vi "hash action stack -- test.vi"() -> ()   [LabVIEW 2012]
uses:
  hash action control.ctl
  stack action -- control.ctl
panel:
  in  "hash action list":T1[](array[typedef])
  out "cursor window action out":T1
  out "stack is empty ?":bool
  in  "hash action":T1
  in  "stack action":T2
  in  "command stack":T1[](array[typedef])
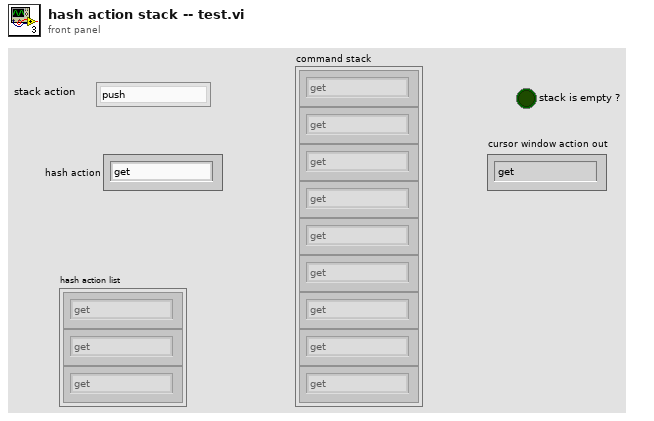
[diagram p1: front panel]
types:
  T1 = typedef "hash action control.ctl" = enum16{"get", "new", "--void"}
  T2 = typedef "stack action -- control.ctl" = enum16{"push", "pop", "check"}
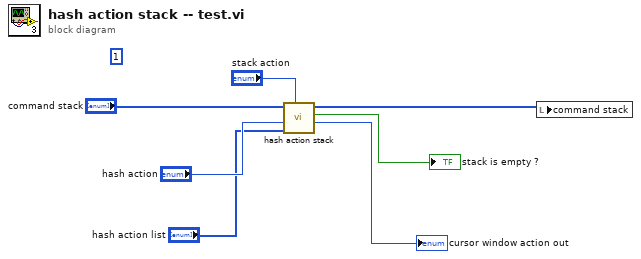
[diagram p0: block diagram]
diagram:
  (unwired) 1
  n1 = call "hash action stack.vi"("stack action"="stack action", "hash action list"="hash action list", "hash action"="hash action", "command stack"="command stack") -> ("cursor window action out"=→"cursor window action out":T1, "stack is empty ?"=→"stack is empty ?":bool, "command stack out"=w6:T1[])  [unwired: 5 in]
  n2 = local write "command stack"(w6) -> ()
